vi "OpenSSH Connect.vi"   [LabVIEW 2020, in "NI_SFTP.lvlib"]
doc: "Connects to an SFTP server using an installed OpenSSH client."
uses:
  <vilib>/net/SFTP/NI_SFTP.lvlib
  <vilib>/net/SSH/Client/OpenSSH/OpenSSH Client.lvclass
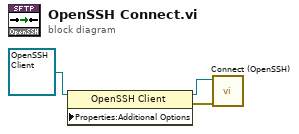
[diagram p0: block diagram]
diagram:
  n1 = property class="OpenSSH Client" props=["Properties:Additional Options"](reference=refnum<class "OpenSSH Client.lvclass"> refnum ("NI_SSH.lvlib:OpenSSH Client")) -> (reference out=w2:refnum<class "OpenSSH Client.lvclass">, error out=w1:errorcluster)  [unwired: 2 in]
  n2 = call <vilib>:"Connect (OpenSSH).vi"("error in"=w1, "client"=w2) -> ()  [unwired: 8 in, 2 out]
